vi "RelayControl.vi"() -> ()   [LabVIEW 2013]
doc: "<B>Motor Control.vi</B> demonstrates simplistic control of a motor using PWM."
uses:
  <vilib>/Rock Robotics/SystemInterfaces/Typedef/FPGA_TypedefDigitalModule.ctl
  <vilib>/Rock Robotics/SystemInterfaces/DIO/FPGA_DIORelayChannel.ctl
  <vilib>/Rock Robotics/WPI/Joystick/WPI_JoystickDeviceEnum.ctl
  Robot_Framework_2014/RollerAction.ctl
panel:
  in  "Relay Channel":T1
  out "Victor LED":bool
  in  "DIO Module":T2
  in  "stop":bool
  # "Wiring Diagram for Digital Sidecar connected to an NI 9403"
  # "Set these inputs before running."
  # "This can be set while running."
  # "Digital Sidecar"
  # "Power\nTerminals"
  # "Motor\nTerminals"
  # "PWM cable"
  # "This shows wiring for a Victor speed controller.  The wiring is similar for a Luminary Micro Jaguar speed controller.  For a Jaguar, you must also select the appropriate instance of the Motor Open VI on the diagram."
  # "V-"
  # "M-"
  # "V+"
  # "M+"
  # "B"
  # "Innovation First"
  # "VICTOR 884"
  # "B"
  # "C"
  # "PWR"
  # "SIG"
  # "(-)"
  # "+V"
  # "10"
  # "9"
  # "8"
  # "7"
  # "6"
  # "5"
  # "4"
  # "3"
  # "2"
  # "1"
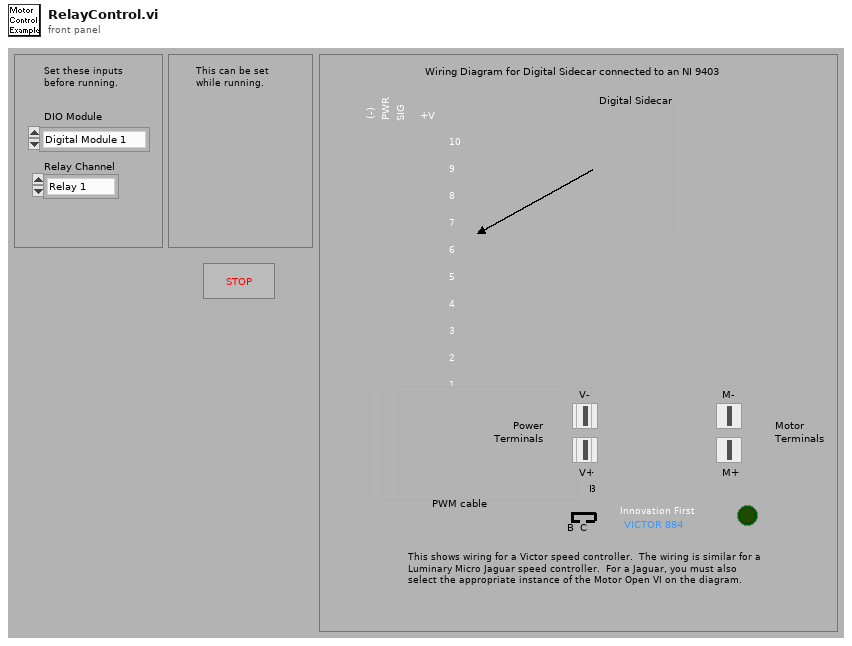
[diagram p1: front panel]
types:
  T1 = typedef "FPGA_DIORelayChannel.ctl" = enum8{"Relay 1", "Relay 2", "Relay 3", "Relay 4", "Relay 5", "Relay 6", "Relay 7", "Relay 8", "Invalid"}
  T2 = typedef "FPGA_TypedefDigitalModule.ctl" = enum16{"Digital Module 1", "Digital Module 2"}
  T3 = typedef "RollerAction.ctl" = enum16{"Init", "Off", "Forward", "Reverse"}
  T4 = typedef "WPI_JoystickDeviceEnum.ctl" = enum16{"USB 1", "USB 2", "USB 3", "USB 4", "Kinect 1", "Kinect 2"}
  T5 = typedef "WPI_RelayDevRef.ctl" = cluster{"DevStatus":errorcluster, "Relay Channel":T1, "Digital Module":T2, "Relay Direction":T6}
  T6 = typedef "WPI_RelayDirection.ctl" = enum16{"Both directions", "Forward only", "Reverse only"}
  T7 = typedef "WPI_JoystickDevRef.ctl" = cluster{"Device":T4}
  T8 = cluster{"axis 1 (x)":dbl, "axis 2 (y)":dbl, "axis 3 (throttle)":dbl, "axis 4":dbl, "axis 5":dbl, "axis 6":dbl}
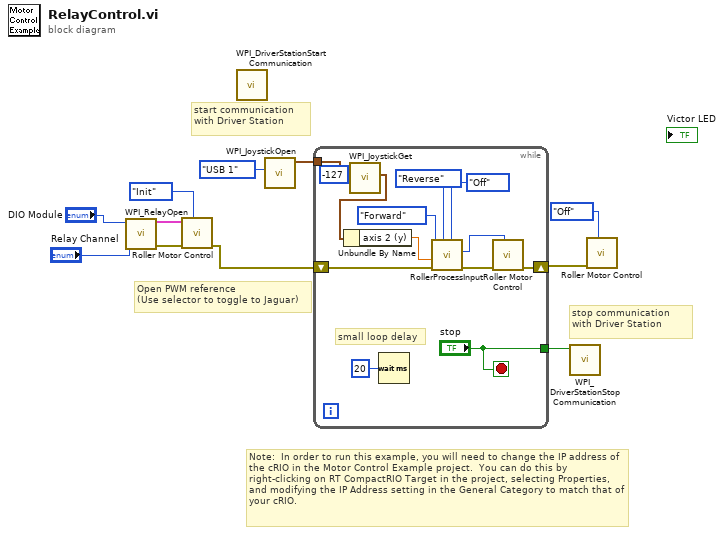
[diagram p0: block diagram]
diagram:
  # "stop communication with Driver Station"
  # "start communication with Driver Station"
  # "Note:  In order to run this example, you will need to change the IP address of the cRIO in the Motor Control Example project.  You can do this by right-clicking on RT CompactRIO Target in the project, selecting Properties, and modifying the IP Address setting in the General Category to match that of your cRIO."
  # "Open PWM reference\n(Use selector to toggle to Jaguar)"
  n1 = call <vilib>:"WPI_RelayOpen.vi"("Relay Channel"="Relay Channel", "Digital Module (Module 1)"="DIO Module") -> ("error out"=w5:errorcluster, "RelayDevRef"=w6:T5)  [unwired: 8 in]
  n2 = call "Roller Motor Control.vi"("Action"=RollerAction."Init", "Error in"=w5, "RelayDevRef"=w6) -> ("Error out"=w3:errorcluster)  [unwired: 8 in]
  n3 = call <vilib>:"WPI_DriverStationStart Communication.vi"() -> ()  [unwired: 1 in, 11 out]
  n4 = call <vilib>:"WPI_JoystickOpen.vi"("JoystickDevice"=WPI_JoystickDeviceEnum."USB 1") -> ("JoystickDevRef"=w9:T7)  [unwired: 10 in]
  n5 = while {
    tunnel: ["stop"] -> w11
    tunnel: w9 -> [w22]
    shift-right: [w20] -> w2
    shift-left: w3 -> [w13]
    stop <- "stop" stop-if-true
    # "small loop delay"
    n6 = call <vilib>:"WPI_JoystickGet.vi"("Scaler"=i8 -127, "JoystickDevRef"=w22) -> ("Axes"=w21:T8)  [unwired: 3 in, 2 out]
    n7 = Unbundle By Name(w21) -> ("axis 2 (y)"=w19:dbl)
    n8 = Wait (ms)(milliseconds to wait=u32 20) -> ()  [unwired: 1 out]
    n9 = call "RollerProcessInput.vi"("OffState"=RollerAction."Off", "ReverseState"=RollerAction."Reverse", "error in"=w13, "JoystickValue"=w19, "ForwardState"=RollerAction."Forward") -> ("error out"=w14:errorcluster, "StateOut"=w15:T3)  [unwired: 5 in]
    n10 = call "Roller Motor Control.vi"("Action"=w15, "Error in"=w14) -> ("Error out"=w20:errorcluster)  [unwired: 9 in]
  }
  n11 = call <vilib>:"WPI_DriverStationStop Communication.vi"("StopCommunication"=w11) -> ()  [unwired: 1 in, 10 out]
  n12 = call "Roller Motor Control.vi"("Action"=RollerAction."Off", "Error in"=w2) -> ()  [unwired: 9 in, 1 out]
